vi "shift_instruction_after.vi"(9 "Sub Offset 2":i32, 10 "PB Instruction":T1, 11 "Subroutines In":T2={"Subroutine A"=[{"Instruct Data"=6, "Op Code"=0, "Flags"=[TRUE, FALSE, FALSE, FALSE, TRUE, TRUE, FALSE, TRUE, FALSE, TRUE, FALSE, FALSE, FALSE, FALSE, FALSE, FALSE, TRUE, TRUE, FALSE, FALSE, FALSE, FALSE, TRUE, FALSE], "Comments"="Blue MOT", "Time (s)"=2.0}, {"Instruct Data"=9, "Op Code"=0, "Flags"=[TRUE, FALSE, FALSE, FALSE, FALSE, TRUE, FALSE, TRUE, FALSE, TRUE, FALSE, FALSE, TRUE, FALSE, FALSE, FALSE, TRUE, TRUE, FALSE, FALSE, FALSE, FALSE, TRUE, FALSE], "Comments"="Hold", "Time (s)"=0.1}, {"Instruct Data"=11, "Op Code"=0, "Flags"=[TRUE, FALSE, FALSE, FALSE, FALSE, FALSE, FALSE, TRUE, FALSE, TRUE, FALSE, FALSE, TRUE, FALSE, FALSE, FALSE, TRUE, TRUE, FALSE, FALSE, FALSE, FALSE, TRUE, FALSE], "Comments"="Repump", "Time (s)"=0.05}, {"Instruct Data"=10, "Op Code"=0, "Flags"=[FALSE, FALSE, FALSE, FALSE, FALSE, TRUE, TRUE, FALSE, TRUE, FALSE, FALSE, TRUE, TRUE, FALSE, FALSE, FALSE, TRUE, FALSE, FALSE, FALSE, FALSE, FALSE, TRUE, FALSE], "Comments"="Red MOT", "Time (s)"=0.2}, {"Instruct Data"=11, "Op Code"=0, "Flags"=[FALSE, FALSE, FALSE, FALSE, FALSE, TRUE, TRUE, FALSE, TRUE, FALSE, FALSE, TRUE, TRUE, FALSE, FALSE, FALSE, FALSE, FALSE, FALSE, FALSE, FALSE, FALSE, TRUE, FALSE], "Comments"="Load ODT", "Time (s)"=0.1}, {"Instruct Data"=11, "Op Code"=0, "Flags"=[FALSE, FALSE, FALSE, FALSE, FALSE, TRUE, TRUE, TRUE, FALSE, FALSE, FALSE, TRUE, TRUE, FALSE, FALSE, FALSE, FALSE, FALSE, FALSE, FALSE, FALSE, FALSE, TRUE, FALSE], "Comments"="ODT Hold", "Time (s)"=0.5}, {"Instruct Data"=11, "Op Code"=0, "Flags"=[FALSE, FALSE, FALSE, FALSE, FALSE, TRUE, TRUE, TRUE, FALSE, FALSE, FALSE, TRUE, TRUE, FALSE, TRUE, FALSE, FALSE, FALSE, FALSE, FALSE, FALSE, FALSE, TRUE, FALSE], "Comments"="", "Time (s)"=0.8}, {"Instruct Data"=200, "Op Code"=2, "Flags"=[FALSE, FALSE, FALSE, FALSE, FALSE, TRUE, TRUE, TRUE, FALSE, FALSE, FALSE, TRUE, TRUE, TRUE, TRUE, FALSE, FALSE, FALSE, FALSE, FALSE, FALSE, TRUE, TRUE, FALSE], "Comments"="loop hold", "Time (s)"=0.01}, {"Instruct Data"=0, "Op Code"=0, "Flags"=[FALSE, FALSE, FALSE, FALSE, FALSE, TRUE, TRUE, TRUE, FALSE, FALSE, FALSE, TRUE, TRUE, TRUE, TRUE, FALSE, FALSE, FALSE, FALSE, FALSE, FALSE, TRUE, TRUE, TRUE], "Comments"="", "Time (s)"=2.5e-06}, {"Instruct Data"=0, "Op Code"=0, "Flags"=[FALSE, FALSE, FALSE, FALSE, FALSE, TRUE, TRUE, TRUE, FALSE, FALSE, FALSE, TRUE, TRUE, TRUE, TRUE, FALSE, FALSE, FALSE, FALSE, FALSE, FALSE, TRUE, TRUE, FALSE], "Comments"="expose uv", "Time (s)"=2e-06}, {"Instruct Data"=7, "Op Code"=3, "Flags"=[FALSE, FALSE, FALSE, FALSE, FALSE, TRUE, TRUE, TRUE, FALSE, FALSE, FALSE, TRUE, TRUE, TRUE, TRUE, FALSE, FALSE, FALSE, FALSE, FALSE, FALSE, TRUE, FALSE, FALSE], "Comments"="", "Time (s)"=1.5e-05}, {"Instruct Data"=0, "Op Code"=0, "Flags"=[FALSE, FALSE, FALSE, FALSE, FALSE, TRUE, TRUE, TRUE, FALSE, FALSE, FALSE, TRUE, TRUE, FALSE, FALSE, FALSE, TRUE, FALSE, FALSE, FALSE, FALSE, TRUE, TRUE, FALSE], "Comments"="Drop", "Time (s)"=0.01}, {"Instruct Data"=0, "Op Code"=0, "Flags"=[FALSE, TRUE, TRUE, TRUE, FALSE, TRUE, TRUE, TRUE, FALSE, FALSE, FALSE, TRUE, TRUE, FALSE, FALSE, FALSE, TRUE, FALSE, FALSE, FALSE, FALSE, FALSE, TRUE, FALSE], "Comments"="Image atoms ", "Time (s)"=1e-05}, {"Instruct Data"=0, "Op Code"=0, "Flags"=[FALSE, FALSE, TRUE, FALSE, FALSE, TRUE, TRUE, TRUE, FALSE, FALSE, FALSE, TRUE, TRUE, FALSE, FALSE, FALSE, TRUE, FALSE, FALSE, FALSE, FALSE, FALSE, TRUE, FALSE], "Comments"="Wait", "Time (s)"=0.081}, {"Instruct Data"=0, "Op Code"=0, "Flags"=[FALSE, TRUE, TRUE, TRUE, FALSE, TRUE, TRUE, TRUE, FALSE, FALSE, FALSE, TRUE, TRUE, FALSE, FALSE, FALSE, TRUE, FALSE, FALSE, FALSE, FALSE, FALSE, TRUE, FALSE], "Comments"="Image BG", "Time (s)"=1e-05}, {"Instruct Data"=0, "Op Code"=6, "Flags"=[FALSE, FALSE, FALSE, FALSE, FALSE, TRUE, TRUE, TRUE, FALSE, FALSE, FALSE, FALSE, TRUE, FALSE, FALSE, FALSE, TRUE, FALSE, FALSE, FALSE, FALSE, FALSE, TRUE, FALSE], "Comments"="Kill time", "Time (s)"=0.5}], "Subroutine B"=[{"Instruct Data"=6, "Op Code"=0, "Flags"=[TRUE, FALSE, FALSE, FALSE, TRUE, TRUE, FALSE, TRUE, FALSE, TRUE, FALSE, FALSE, FALSE, FALSE, FALSE, FALSE, TRUE, TRUE, FALSE, FALSE, FALSE, FALSE, TRUE, FALSE], "Comments"="Blue MOT", "Time (s)"=2.0}, {"Instruct Data"=9, "Op Code"=0, "Flags"=[TRUE, FALSE, FALSE, FALSE, FALSE, TRUE, FALSE, TRUE, FALSE, TRUE, FALSE, FALSE, TRUE, FALSE, FALSE, FALSE, TRUE, TRUE, FALSE, FALSE, FALSE, FALSE, TRUE, FALSE], "Comments"="Hold", "Time (s)"=0.1}, {"Instruct Data"=11, "Op Code"=0, "Flags"=[TRUE, FALSE, FALSE, FALSE, FALSE, FALSE, FALSE, TRUE, FALSE, TRUE, FALSE, FALSE, TRUE, FALSE, FALSE, FALSE, TRUE, TRUE, FALSE, FALSE, FALSE, FALSE, TRUE, FALSE], "Comments"="Repump", "Time (s)"=0.05}, {"Instruct Data"=10, "Op Code"=0, "Flags"=[FALSE, FALSE, FALSE, FALSE, FALSE, TRUE, TRUE, FALSE, TRUE, FALSE, FALSE, TRUE, TRUE, FALSE, FALSE, FALSE, TRUE, FALSE, FALSE, FALSE, FALSE, FALSE, TRUE, FALSE], "Comments"="Red MOT", "Time (s)"=0.2}, {"Instruct Data"=11, "Op Code"=0, "Flags"=[FALSE, FALSE, FALSE, FALSE, FALSE, TRUE, TRUE, FALSE, TRUE, FALSE, FALSE, TRUE, TRUE, FALSE, FALSE, FALSE, FALSE, FALSE, FALSE, FALSE, FALSE, FALSE, TRUE, FALSE], "Comments"="Load ODT", "Time (s)"=0.1}, {"Instruct Data"=11, "Op Code"=0, "Flags"=[FALSE, FALSE, FALSE, FALSE, FALSE, TRUE, TRUE, TRUE, FALSE, FALSE, FALSE, TRUE, TRUE, FALSE, FALSE, FALSE, FALSE, FALSE, FALSE, FALSE, FALSE, FALSE, TRUE, FALSE], "Comments"="ODT Hold", "Time (s)"=0.5}, {"Instruct Data"=11, "Op Code"=0, "Flags"=[FALSE, FALSE, FALSE, FALSE, FALSE, TRUE, TRUE, TRUE, FALSE, FALSE, FALSE, TRUE, TRUE, FALSE, TRUE, FALSE, FALSE, FALSE, FALSE, FALSE, FALSE, FALSE, TRUE, FALSE], "Comments"="", "Time (s)"=0.8}, {"Instruct Data"=200, "Op Code"=2, "Flags"=[FALSE, FALSE, FALSE, FALSE, FALSE, TRUE, TRUE, TRUE, FALSE, FALSE, FALSE, TRUE, TRUE, TRUE, TRUE, FALSE, FALSE, FALSE, FALSE, FALSE, FALSE, TRUE, TRUE, FALSE], "Comments"="loop hold", "Time (s)"=0.01}, {"Instruct Data"=0, "Op Code"=0, "Flags"=[FALSE, FALSE, FALSE, FALSE, FALSE, TRUE, TRUE, TRUE, FALSE, FALSE, FALSE, TRUE, TRUE, TRUE, TRUE, FALSE, FALSE, FALSE, FALSE, FALSE, FALSE, TRUE, TRUE, TRUE], "Comments"="", "Time (s)"=2.5e-06}, {"Instruct Data"=0, "Op Code"=0, "Flags"=[FALSE, FALSE, FALSE, FALSE, FALSE, TRUE, TRUE, TRUE, FALSE, FALSE, FALSE, TRUE, TRUE, TRUE, TRUE, FALSE, FALSE, FALSE, FALSE, FALSE, FALSE, TRUE, TRUE, FALSE], "Comments"="expose uv", "Time (s)"=2e-06}, {"Instruct Data"=7, "Op Code"=3, "Flags"=[FALSE, FALSE, FALSE, FALSE, FALSE, TRUE, TRUE, TRUE, FALSE, FALSE, FALSE, TRUE, TRUE, TRUE, TRUE, FALSE, FALSE, FALSE, FALSE, FALSE, FALSE, TRUE, FALSE, FALSE], "Comments"="", "Time (s)"=1.5e-05}, {"Instruct Data"=0, "Op Code"=0, "Flags"=[FALSE, FALSE, FALSE, FALSE, FALSE, TRUE, TRUE, TRUE, FALSE, FALSE, FALSE, TRUE, TRUE, FALSE, FALSE, FALSE, TRUE, FALSE, FALSE, FALSE, FALSE, TRUE, TRUE, FALSE], "Comments"="Drop", "Time (s)"=0.01}, {"Instruct Data"=0, "Op Code"=0, "Flags"=[FALSE, TRUE, TRUE, TRUE, FALSE, TRUE, TRUE, TRUE, FALSE, FALSE, FALSE, TRUE, TRUE, FALSE, FALSE, FALSE, TRUE, FALSE, FALSE, FALSE, FALSE, FALSE, TRUE, FALSE], "Comments"="Image atoms ", "Time (s)"=1e-05}, {"Instruct Data"=0, "Op Code"=0, "Flags"=[FALSE, FALSE, TRUE, FALSE, FALSE, TRUE, TRUE, TRUE, FALSE, FALSE, FALSE, TRUE, TRUE, FALSE, FALSE, FALSE, TRUE, FALSE, FALSE, FALSE, FALSE, FALSE, TRUE, FALSE], "Comments"="Wait", "Time (s)"=0.081}, {"Instruct Data"=0, "Op Code"=0, "Flags"=[FALSE, TRUE, TRUE, TRUE, FALSE, TRUE, TRUE, TRUE, FALSE, FALSE, FALSE, TRUE, TRUE, FALSE, FALSE, FALSE, TRUE, FALSE, FALSE, FALSE, FALSE, FALSE, TRUE, FALSE], "Comments"="Image BG", "Time (s)"=1e-05}, {"Instruct Data"=0, "Op Code"=6, "Flags"=[FALSE, FALSE, FALSE, FALSE, FALSE, TRUE, TRUE, TRUE, FALSE, FALSE, FALSE, FALSE, TRUE, FALSE, FALSE, FALSE, TRUE, FALSE, FALSE, FALSE, FALSE, FALSE, TRUE, FALSE], "Comments"="Kill time", "Time (s)"=0.5}], "Interleave On"=FALSE, "Number of loops"=0, "Insert after instruction"=0} {"Insert after instruction" min=0; "Subroutine B"."Time (s)" min=5e-08 format="%.3p"; "Subroutine B"."Op Code" items=["Continue", "Stop", "Loop", "End Loop", "JSR", "RTS", "Branch", "Long Delay", "Wait"]; "Subroutine B"."Instruct Data" format="%.0p"; "Subroutine A"."Time (s)" min=5e-08 format="%.3p"; "Subroutine A"."Op Code" items=["Continue", "Stop", "Loop", "End Loop", "JSR", "RTS", "Branch", "Long Delay", "Wait"]; "Subroutine A"."Instruct Data" format="%.0p"}) -> (2 "Instruction Out":T1)   [LabVIEW 2013]
uses:
  Controls/PulseBlaster/interleaveControls.ctl
panel:
  in  "Sub Offset 3":i32
  # "1"
  # "2"
  # "3"
  # "4"
  # "5"
  # "6"
  # "7"
  # "8"
  # "9"
  # "10"
  # "11"
  # "12"
  # "13"
  # "14"
  # "15"
  # "16"
  # "17"
  # "18"
  # "19"
  # "20"
  # "21"
  # "22"
  # "23"
  # "24"
  # "1"
  # "2"
  # "3"
  # "4"
  # "5"
  # "6"
  # "7"
  # "8"
  # "9"
  # "10"
  # "11"
  # "12"
  # "13"
  # "14"
  # "15"
  # "16"
  # "17"
  # "18"
  # "19"
  # "20"
  # "21"
  # "22"
  # "23"
  # "24"
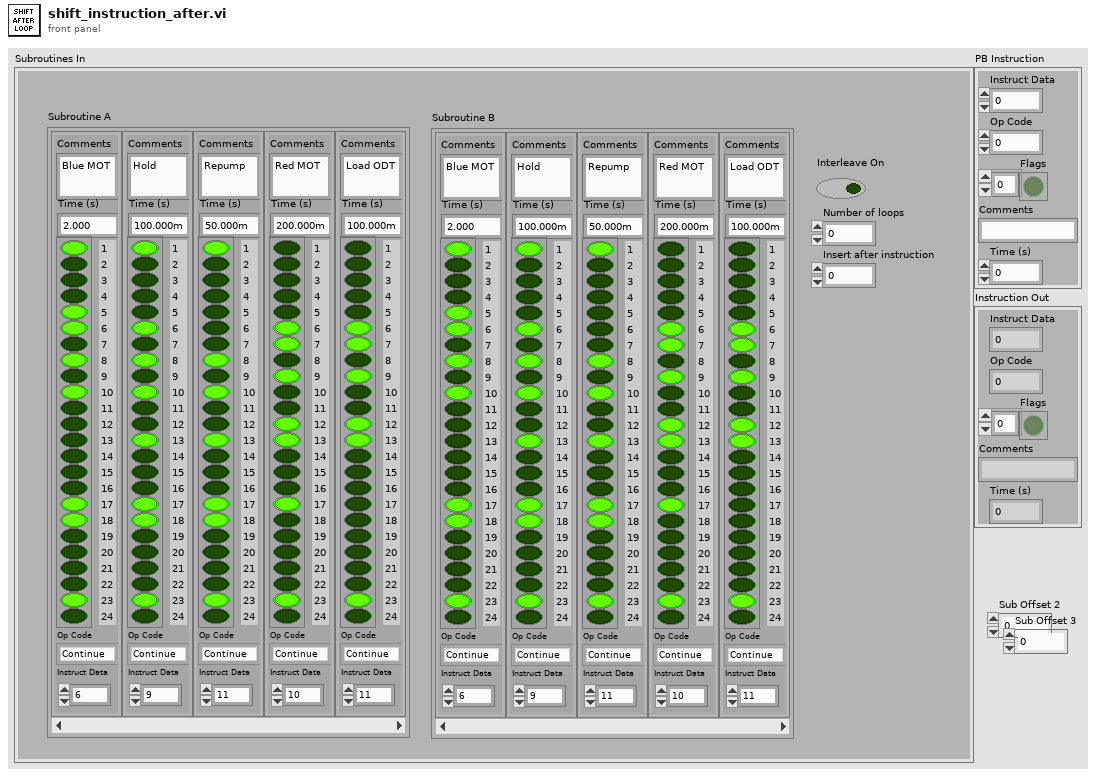
[diagram p1: front panel]
types:
  T1 = cluster{"Instruct Data":i32, "Op Code":i32, "Flags":bool[], "Comments":string, "Time (s)":dbl}
  T2 = typedef "interleaveControls.ctl" = cluster{"Subroutine A":cluster{"Instruct Data":i32, "Op Code":i32, "Flags":bool[], "Comments":string, "Time (s)":dbl}[], "Subroutine B":cluster{"Instruct Data":i32, "Op Code":i32, "Flags":bool[], "Comments":string, "Time (s)":dbl}[], "Interleave On":bool, "Number of loops":i32, "Insert after instruction":i32}
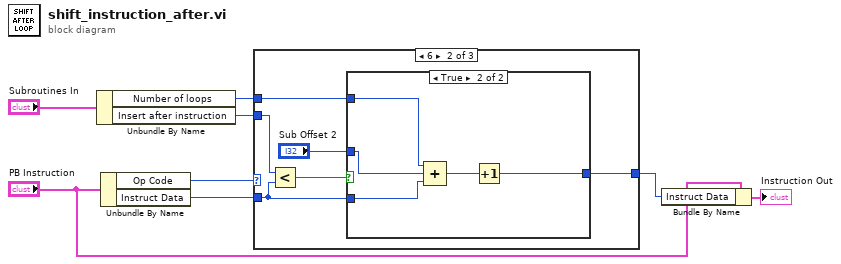
[diagram p0: block diagram]
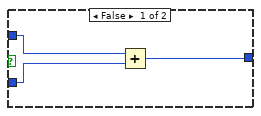
[diagram p3: hidden frame]
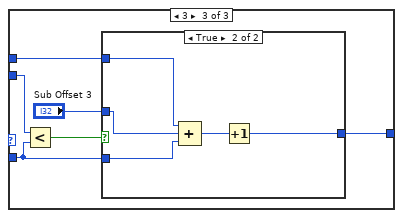
[diagram p4: hidden frame]
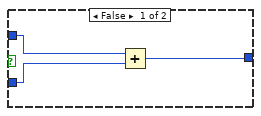
[diagram p5: hidden frame]
diagram:
  n1 = Unbundle By Name("Subroutines In") -> ("Number of loops"=w4:i32, "Insert after instruction"=w5:i32)
  n2 = Unbundle By Name("PB Instruction") -> ("Op Code"=w7:i32, "Instruct Data"=w6:i32)
  n3 = case shown="6" w7 {
    tunnel: w6 -> [w9 w11 w25]
    tunnel: w5 -> [_ w15 w29]
    tunnel: w4 -> [_ w13 w27]
    tunnel: [w9 w10 w24] -> w1
    frame 0, Default {
    }
    frame 6 {
      n4 = Less?(x=w15, y=w11) -> (x < y?=w14:bool)
      n5 = case shown="True" w14 {
        tunnel: w13 -> [_ w23]
        tunnel: "Sub Offset 2" -> [w18 w22]
        tunnel: w11 -> [w17 w21]
        tunnel: [w16 w19] -> w10
        frame False {
          n6 = Add(x=w18, y=w17) -> (x+y=w16:i32)
        }
        frame True {
          n7 = Compound Arithmetic op=ADD(w23, w22, w21) -> (w20:i32)
          n8 = Increment(x=w20) -> (x+1=w19:i32)
        }
      }
    }
    frame 3 {
      n9 = Less?(x=w29, y=w25) -> (x < y?=w28:bool)
      n10 = case shown="True" w28 {
        tunnel: w27 -> [_ w37]
        tunnel: "Sub Offset 3" -> [w32 w36]
        tunnel: w25 -> [w31 w35]
        tunnel: [w30 w33] -> w24
        frame False {
          n11 = Add(x=w32, y=w31) -> (x+y=w30:i32)
        }
        frame True {
          n12 = Compound Arithmetic op=ADD(w37, w36, w35) -> (w34:i32)
          n13 = Increment(x=w34) -> (x+1=w33:i32)
        }
      }
    }
  }
  n14 = Bundle By Name(cluster="PB Instruction", "Instruct Data"=w1) -> (→"Instruction Out":T1)
